vi "Create.vi"(8 "error in (no error)":errorcluster, 10 "Input":string) -> (0 "error out":errorcluster, 3 "Hailstone Out":refnum<class "Vector.lvclass">)   [LabVIEW 2021, in "Vector.lvclass"]
uses:
  Vector.lvclass
  Vector.lvclass/Vector.ctl
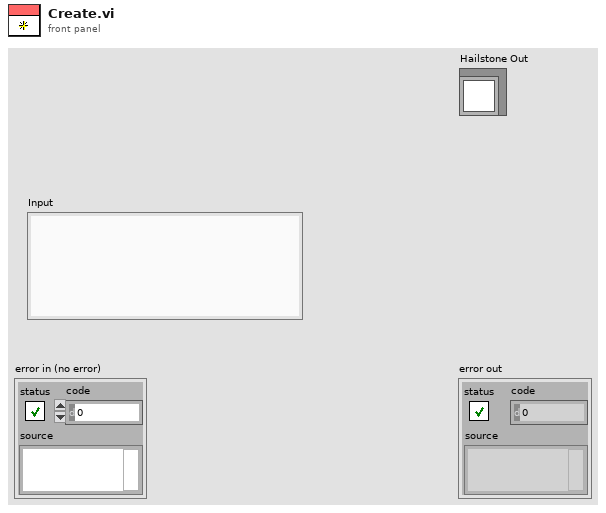
[diagram p1: front panel]
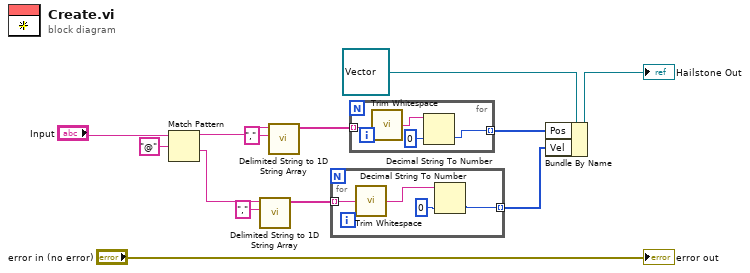
[diagram p0: block diagram]
diagram:
  n1 = Match Pattern(string="Input", regular expression="@") -> (before substring=w9:string, after substring=w8:string)  [unwired: 1 in, 2 out]
  n2 = call <vilib>:"Delimited String to 1D String Array.vi"("delimiter"=",", "delimited string"=w8) -> ("string array"=w5:string[])  [unwired: 9 in]
  n3 = call <vilib>:"Delimited String to 1D String Array.vi"("delimiter"=",", "delimited string"=w9) -> ("string array"=w4:string[])  [unwired: 9 in]
  n4 = for {
    tunnel: w5 -> [w17] mode=indexing
    tunnel: [w14] -> w1 mode=indexing
    n5 = call <vilib>:"Trim Whitespace.vi"("string"=w17) -> ("trimmed string"=w16:string)  [unwired: 1 in]
    n6 = Decimal String To Number(string=w16, default (0L)=i64 0 ("default (0 DBL)")) -> (number=w14:i64)  [unwired: 1 in, 1 out]
  }
  n7 = for {
    tunnel: w4 -> [w21] mode=indexing
    tunnel: [w18] -> w2 mode=indexing
    n8 = call <vilib>:"Trim Whitespace.vi"("string"=w21) -> ("trimmed string"=w20:string)  [unwired: 1 in]
    n9 = Decimal String To Number(string=w20, default (0L)=i64 0 ("default (0 DBL)")) -> (number=w18:i64)  [unwired: 1 in, 1 out]
  }
  n10 = Bundle By Name(cluster=refnum<class "Vector.lvclass"> refnum ("Proto"), "Pos"=w2, "Vel"=w1) -> (→"Hailstone Out":refnum<class "Vector.lvclass">)
  "error out" <- "error in (no error)"
